vi "Emit Beep.vi"(7 "Enable Beep (F)":bool, 8 "error in (no error)":errorcluster, 9 "Beep Duration (.25 s)":dbl=0.25, 10 "Beep Frequency (300)":dbl=300.0, 11 "VISA resource name":refnum<visa-resource-name>) -> (0 "error out":errorcluster, 3 "VISA resource name out":refnum<visa-resource-name>)   [LabVIEW 2019, in "Keithley 24XX.lvlib"]
doc: "Emits a beep of a user defined frequency and duration."
uses:
  <instrlib>/Keithley 24XX/Keithley 24XX.lvlib
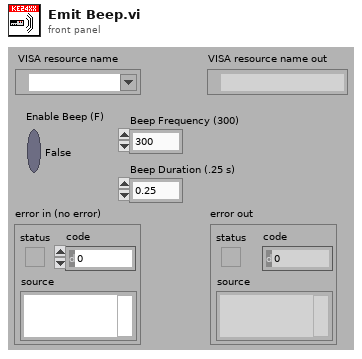
[diagram p1: front panel]
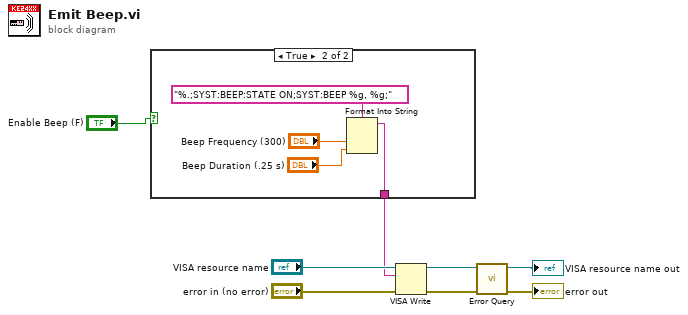
[diagram p0: block diagram]
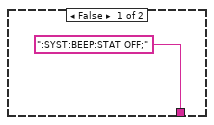
[diagram p2: hidden frame]
diagram:
  n1 = case shown="True" "Enable Beep (F)" {
    tunnel: [":SYST:BEEP:STAT OFF;" w13] -> w2
    frame False {
    }
    frame True {
      n2 = Format Into String(format string="%.;SYST:BEEP:STATE ON;SYST:BEEP %g, %g;", "Beep Frequency (300)", "Beep Duration (.25 s)") -> (resulting string=w13:string)  [unwired: 2 in, 1 out]
    }
  }
  n3 = VISA Write(VISA resource name="VISA resource name", write buffer=w2, error in (no error)="error in (no error)") -> (VISA resource name out=w6:refnum<visa-resource-name>, error out=w3:errorcluster)  [unwired: 1 out]
  n4 = call <instrlib>:"Error Query.vi"("error in (no error)"=w3, "VISA resource name"=w6) -> ("error out"=→"error out":errorcluster, "VISA resource name out"=→"VISA resource name out":refnum<visa-resource-name>)  [unwired: 6 in, 2 out]
